vi "clignotant.vi"() -> ()   [LabVIEW 2025]
panel:
  in  "sw":bool
  out "led":bool
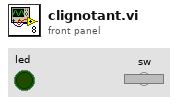
[diagram p1: front panel]
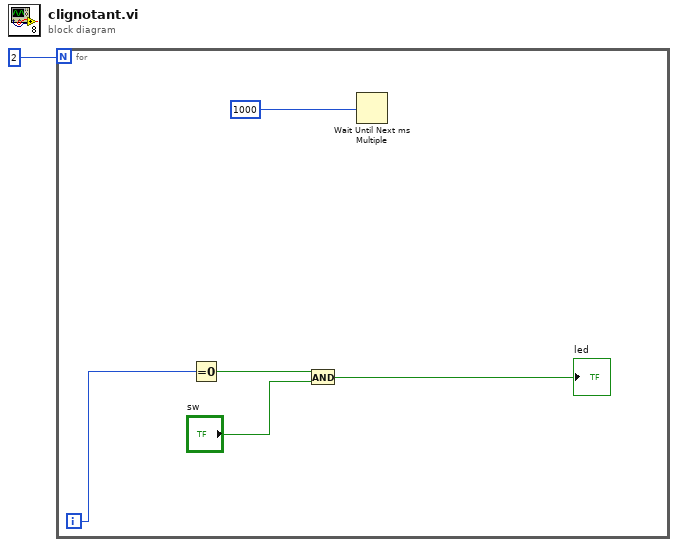
[diagram p0: block diagram]
diagram:
  n1 = for {
    N: 2 -> [_]
    i -> [w5]
    n2 = Equal To 0?(x=w5) -> (x = 0?=w4:bool)
    n3 = And(x=w4, y="sw") -> (x .and. y?=→"led":bool)
    n4 = Wait Until Next ms Multiple(millisecond multiple=1000) -> ()  [unwired: 1 out]
  }
